vi "MapEqualScale.vi"(8 "error in (no error)":errorcluster, 11 "reference":refnum<vi>) -> (0 "error out":errorcluster, 3 "reference out":refnum<vi>)   [LabVIEW 2014]
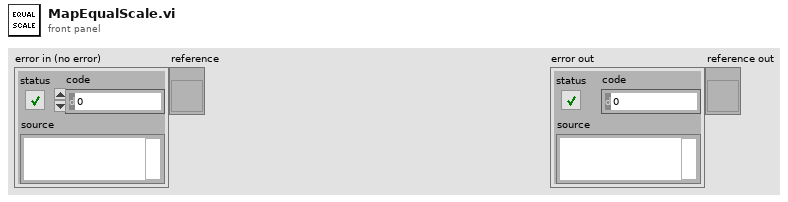
[diagram p1: front panel]
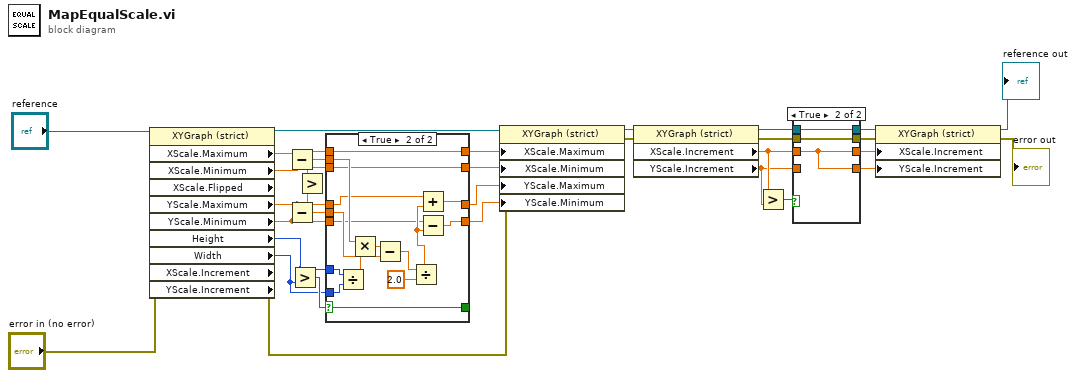
[diagram p0: block diagram]
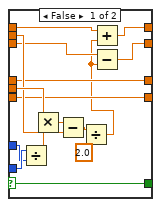
[diagram p3: hidden frame]
diagram:
  n1 = property class="XYGraph (strict)" props=["XScale", "Maximum", "XScale", "Minimum", "XScale", "Flipped", "YScale", "Maximum", "YScale", "Minimum", "Height", "Width", "XScale", "Increment", "YScale", "Increment"](reference="reference", error in="error in (no error)") -> (reference out=w30:refnum<vi>, error out=w16:errorcluster, "XScale.Maximum"=w27:dbl, "XScale.Minimum"=w25:dbl, "YScale.Maximum"=w24:dbl, "YScale.Minimum"=w22:dbl, "Height"=w28:u32, "Width"=w17:u32)  [unwired: 3 out]
  n2 = Subtract(x=w27, y=w25) -> (x-y=w26:dbl)
  n3 = Subtract(x=w24, y=w22) -> (x-y=w23:dbl)
  n4 = Greater?(x=w28, y=w17) -> (0:w29:bool)
  n5 = Greater?(x=w26, y=w23) -> ()  [unwired: 1 out]
  n6 = case shown="True" w29 {
    selector: w29 -> [w31 w57]
    tunnel: w17 -> [w46 w48]
    tunnel: w28 -> [w45 w47]
    tunnel: w27 -> [w40 w51]
    tunnel: w26 -> [w41 w59]
    tunnel: w25 -> [w39 w52]
    tunnel: w24 -> [w36 w50]
    tunnel: w23 -> [w43 w58]
    tunnel: w22 -> [w35 w49]
    tunnel: [w38 w51] -> w21
    tunnel: [w37 w52] -> w20
    tunnel: [w36 w54] -> w19
    tunnel: [w35 w53] -> w18
    tunnel: [w31 w57] -> _
    frame False {
      n7 = Divide(x=w46, y=w45) -> (x/y=w44:dbl)
      n8 = Multiply(x=w43, y=w44) -> (x*y=w42:dbl)
      n9 = Subtract(x=w42, y=w41) -> (x-y=w34:dbl)
      n10 = Divide(x=w34, y=2.0) -> (x/y=w32:dbl)
      n11 = Add(x=w40, y=w32) -> (x+y=w38:dbl)
      n12 = Subtract(x=w39, y=w32) -> (x-y=w37:dbl)
    }
    frame True {
      n13 = Divide(x=w47, y=w48) -> (x/y=w62:dbl)
      n14 = Multiply(x=w59, y=w62) -> (x*y=w61:dbl)
      n15 = Subtract(x=w61, y=w58) -> (x-y=w60:dbl)
      n16 = Divide(x=w60, y=2.0) -> (x/y=w56:dbl)
      n17 = Add(x=w50, y=w56) -> (x+y=w54:dbl)
      n18 = Subtract(x=w49, y=w56) -> (x-y=w53:dbl)
    }
  }
  n19 = property class="XYGraph (strict)"(reference=w30, error in=w16, "XScale.Maximum"=w21, "XScale.Minimum"=w20, "YScale.Maximum"=w19, "YScale.Minimum"=w18) -> (reference out=w15:refnum<vi>, error out=w12:errorcluster)
  n20 = property class="XYGraph (strict)"(reference=w15, error in=w12) -> (reference out=w10:refnum<vi>, error out=w11:errorcluster, "XScale.Increment"=w3:dbl, "YScale.Increment"=w2:dbl)
  n21 = Greater?(x=w3, y=w2) -> (0:w1:bool)
  n22 = case shown="True" w1 {
    tunnel: w11 -> [w64 w67]
    tunnel: w10 -> [w65 w68]
    tunnel: [w65 w68] -> w9
    tunnel: [w64 w67] -> w8
    tunnel: [w63 w66] -> w7
    tunnel: w3 -> [_ w66]
    tunnel: [w63 w66] -> w6
    tunnel: w2 -> [w63 _]
    frame False {
    }
    frame True {
    }
  }
  n23 = property class="XYGraph (strict)"(reference=w9, error in=w8, "XScale.Increment"=w7, "YScale.Increment"=w6) -> (reference out=→"reference out":refnum<vi>, error out=→"error out":errorcluster)
